vi "createNotifier.vi"(8 "error in (no error)":errorcluster, 11 "TcpServer in":refnum<class "TcpServer.lvclass">) -> (0 "error out":errorcluster, 3 "TcpServer out":refnum<class "TcpServer.lvclass">)   [LabVIEW 2018, in "TcpServer.lvclass"]
doc: "Create notifier reference to stop a process runing in runServer.vi."
uses:
  TcpServer.lvclass
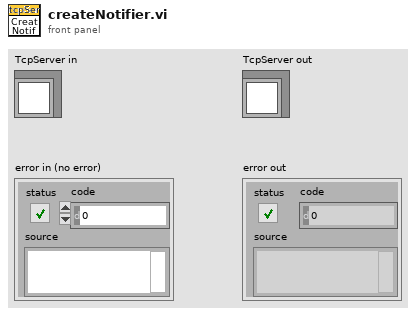
[diagram p1: front panel]
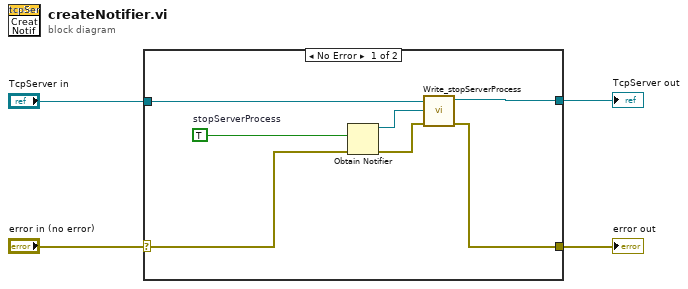
[diagram p0: block diagram]
diagram:
  n1 = case shown="No Error" "error in (no error)" {
    selector: "error in (no error)" -> [w10 w12]
    tunnel: [w6 w12] -> w3
    tunnel: "TcpServer in" -> [w8 w13]
    tunnel: [w5 w13] -> w1
    frame No Error {
      w11 = TRUE  # stopServerProcess
      n2 = Obtain Notifier(notification data type=w11, error in (no error)=w10) -> (notifier out=w9:refnum<notifier>, error out=w7:errorcluster)  [unwired: 2 in, 1 out]
      n3 = call-dynamic "Write_stopServerProcess.vi"("error in (no error)"=w7, "stopServerProcess"=w9, "TcpServer in"=w8) -> ("error out"=w6:errorcluster, "TcpServer out"=w5:refnum<class "TcpServer.lvclass">)  [unwired: 7 in]
    }
    frame Error {
    }
  }
  "error out" <- w3
  "TcpServer out" <- w1
